vi "Read Header.vi"(8 "error in (no error)":errorcluster, 11 "CIFfifo in":refnum<class "CIFfifo.lvclass">) -> (0 "error out":errorcluster, 2 "Header":T1, 3 "CIFfifo out":refnum<class "CIFfifo.lvclass">)   [LabVIEW 2021, in "CIFfifo.lvclass"]
uses:
  CIFfifo.lvclass
  typedef/FIFO Header.ctl
  CIFfifo.lvclass/CIFfifo.ctl
  ChannelCommon.lvlib
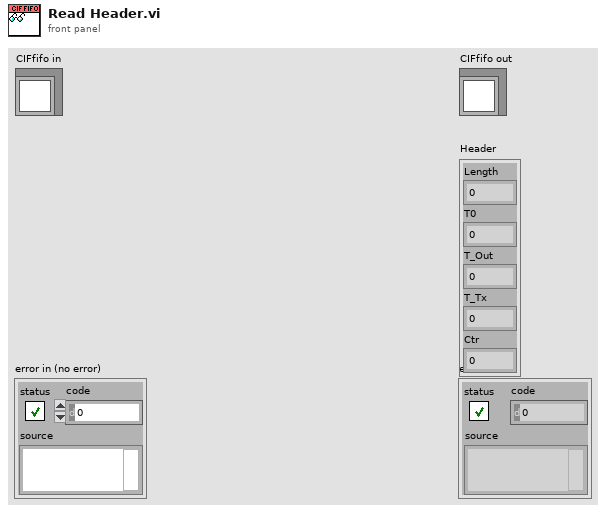
[diagram p1: front panel]
types:
  T1 = typedef "ChannelCommon.lvlib/FIFO Header.ctl" = cluster{"Length":u64, "T0":u64, "T_Out":u64, "T_Tx":u64, "Ctr":u64}
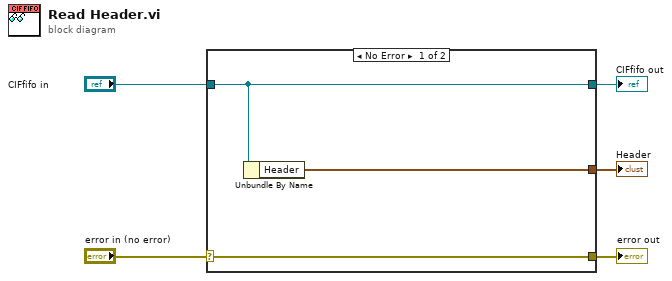
[diagram p0: block diagram]
diagram:
  n1 = case shown="No Error" "error in (no error)" {
    selector: "error in (no error)" -> [w8 w9]
    tunnel: [w8 w9] -> w4
    tunnel: [w7 w10] -> w2
    tunnel: "CIFfifo in" -> [w7 w10]
    tunnel: [w6 _] -> w1
    frame No Error {
      n2 = Unbundle By Name(w7) -> ("Header"=w6:T1)
    }
    frame Error {
    }
  }
  "error out" <- w4
  "CIFfifo out" <- w2
  "Header" <- w1
